vi "0037-Sub_map_meas.vi"(6 "数値":dbl, 7 "温湿度データ":dbl[][](array[numeric]), 8 "error out":errorcluster, 11 "device":T1) -> (0 "error out 2":errorcluster caption="error out", 2 "出力配列":dbl[](array[numeric]), 3 "device 2":T1, 4 "配列":bool[](array[boolean]), 5 "温湿度データ 2":dbl[][](array[numeric]))   [LabVIEW 2014]
uses:
  LV-CP2112_2014/LVProject/private/CP2112_device.ctl
  LV-CP2112_2014/LVProject/private/CP2112_SMBUS_S0.ctl
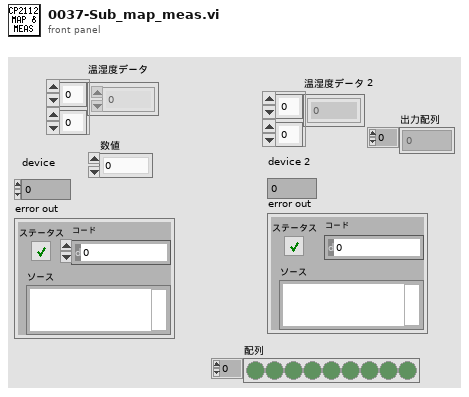
[diagram p1: front panel]
types:
  T1 = typedef "CP2112_device.ctl" = i32
  T2 = typedef "CP2112_SMBUS_S0.ctl" = enum8{"HID_SMBUS_S0_IDLE", "HID_SMBUS_S0_BUSY", "HID_SMBUS_S0_COMPLETE", "HID_SMBUS_S0_ERROR"}
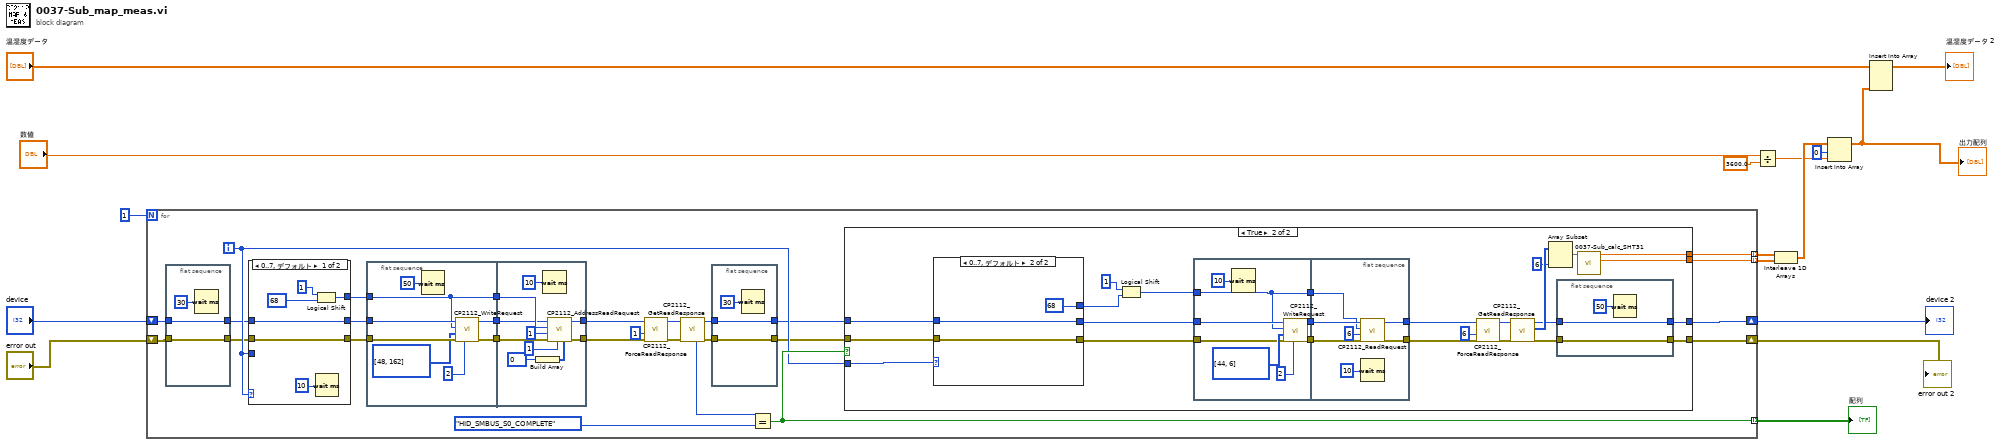
[diagram p0: block diagram]
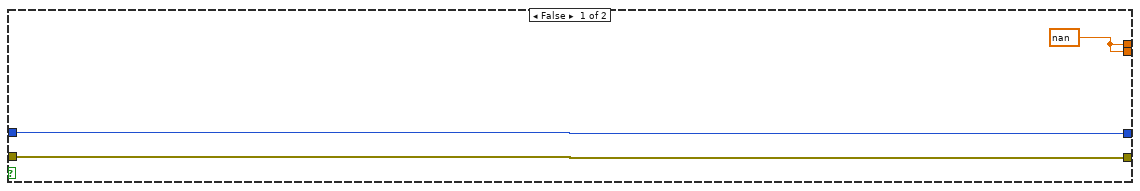
[diagram p2: hidden frame]
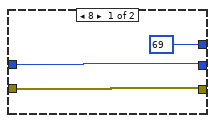
[diagram p3: hidden frame]
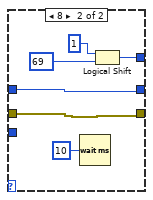
[diagram p4: hidden frame]
diagram:
  n1 = for {
    N: 1 -> [_]
    shift-right: [w28] -> w15
    shift-left: "error out" -> [w20]
    shift-right: [w29] -> w16
    shift-left: "device" -> [w19]
    tunnel: [w30] -> w13 mode=indexing
    tunnel: [w26] -> w8 mode=indexing
    tunnel: [w25] -> w7 mode=indexing
    i -> [w27]
    n2 = flat-sequence {
      tunnel: [w46] -> w18
      tunnel: w19 -> [w46]
      tunnel: [w45] -> w17
      tunnel: w20 -> [w45]
      frame #0 {
        n3 = Wait (ms)(milliseconds to wait=u32 30 ("ミリ秒待機時間")) -> ()  [unwired: 1 out]
      }
    }
    n4 = case shown="0..7, デフォルト" w27 {
      tunnel: [w123 w130] -> w36
      tunnel: w17 -> [w121 w127]
      tunnel: [w121 w127] -> w37
      tunnel: w18 -> [w120 w126]
      tunnel: [w120 w126] -> w38
      tunnel: w27 -> [_ _]
      frame 0..7, Default {
        n5 = Logical Shift(y=1, x=68) -> (x << y=w123:i32)
        n6 = Wait (ms)(milliseconds to wait=u32 10 ("ミリ秒待機時間")) -> ()  [unwired: 1 out]
      }
      frame 8 {
        n7 = Wait (ms)(milliseconds to wait=u32 10 ("ミリ秒待機時間")) -> ()  [unwired: 1 out]
        n8 = Logical Shift(y=1, x=69) -> (x << y=w130:i32)
      }
    }
    n9 = flat-sequence {
      tunnel: w38 -> [w109]
      tunnel: w37 -> [w107]
      tunnel: w36 -> [w105]
      tunnel: [w108] -> w35
      tunnel: [w106] -> w34
      tunnel: [w105] -> w33
      tunnel: w35 -> [w114]
      tunnel: w34 -> [w113]
      tunnel: w33 -> [w115]
      tunnel: [w112] -> w32
      tunnel: [w111] -> w31
      frame #0 {
        n10 = Wait (ms)(milliseconds to wait=u32 50 ("ミリ秒待機時間")) -> ()  [unwired: 1 out]
        n11 = call "CP2112_WriteRequest.vi"("numBytesToWrite"=u8 2, "error in (no error)"=w107, "buffer"=u8[] [48, 162], "slaveAddress"=w105, "device"=w109) -> ("error out"=w106:errorcluster, "deviceOut"=w108:T1)  [unwired: 4 in, 1 out]
      }
      frame #1 {
        n12 = Build Array(u8 0 ("targetAddressSize")) -> (w118:u8[])
        n13 = Wait (ms)(milliseconds to wait=u32 10 ("ミリ秒待機時間")) -> ()  [unwired: 1 out]
        n14 = call "CP2112_AddressReadRequest.vi"("targetAddress[]"=w118, "targetAddressSize"=u8 1, "error in (no error)"=w113, "numByteToRead"=i16 1, "slaveAddress"=w115, "device"=w114) -> ("error out"=w112:errorcluster, "deviceOut"=w111:T1)  [unwired: 3 in, 1 out]
      }
    }
    n15 = call "CP2112_ForceReadResponse.vi"("error in (no error)"=w32, "numByteToRead"=i16 1, "device"=w31) -> ("error out"=w43:errorcluster, "deviceOut"=w42:T1)  [unwired: 6 in, 1 out]
    n16 = call "CP2112_GetReadResponse.vi"("error in (no error)"=w43, "device"=w42) -> ("error out"=w21:errorcluster, "deviceOut"=w23:T1, "HID_SMBUS_S0"=w39:T2)  [unwired: 4 in, 3 out]
    n17 = flat-sequence {
      tunnel: [w49] -> w24
      tunnel: w23 -> [w49]
      tunnel: [w48] -> w22
      tunnel: w21 -> [w48]
      frame #0 {
        n18 = Wait (ms)(milliseconds to wait=u32 30 ("ミリ秒待機時間")) -> ()  [unwired: 1 out]
      }
    }
    n19 = Equal?(x=w39, y=CP2112_SMBUS_S0."HID_SMBUS_S0_COMPLETE" ("HID_SMBUS_S0")) -> (x = y?=w30:bool)
    n20 = case shown="TRUE" w30 {
      tunnel: [w51 w55] -> w28
      tunnel: [w52 w57] -> w29
      tunnel: w24 -> [w52 w72]
      tunnel: w22 -> [w51 w71]
      tunnel: w27 -> [_ w53]
      tunnel: [w50 w69] -> w26
      tunnel: [w50 w68] -> w25
      frame False {
        w50 = nan ("新規要素/部分配列")
      }
      frame True {
        n21 = case shown="0..7, デフォルト" w53 {
          tunnel: [w96 w100] -> w63
          tunnel: [w97 w99] -> w64
          tunnel: [u32 69 ("ミリ秒待機時間") u32 68 ("ミリ秒待機時間")] -> w66
          tunnel: w72 -> [w97 w99]
          tunnel: w71 -> [w96 w100]
          frame 8 {
          }
          frame 0..7, Default {
          }
        }
        n22 = Logical Shift(y=1, x=w66) -> (x << y=w65:u32)
        n23 = flat-sequence {
          tunnel: w65 -> [w82]
          tunnel: w64 -> [w84]
          tunnel: w63 -> [w83]
          tunnel: [w88] -> w62
          tunnel: [w87] -> w61
          tunnel: [w82] -> w58
          tunnel: w62 -> [w90]
          tunnel: w61 -> [w92]
          tunnel: [w94] -> w60
          tunnel: [w93] -> w59
          tunnel: w58 -> [w91]
          frame #0 {
            n24 = Wait (ms)(milliseconds to wait=u32 10 ("ミリ秒待機時間")) -> ()  [unwired: 1 out]
            n25 = call "CP2112_WriteRequest.vi"("numBytesToWrite"=i16 2 ("numByteToRead"), "error in (no error)"=w83, "buffer"=u8[] [44, 6], "slaveAddress"=w82, "device"=w84) -> ("error out"=w88:errorcluster, "deviceOut"=w87:T1)  [unwired: 4 in, 1 out]
          }
          frame #1 {
            n26 = call "CP2112_ReadRequest.vi"("error in (no error)"=w90, "numByteToRead"=i16 6, "slaveAddress"=w91, "device"=w92) -> ("error out"=w94:errorcluster, "deviceOut"=w93:T1)  [unwired: 5 in, 1 out]
            n27 = Wait (ms)(milliseconds to wait=u32 10 ("ミリ秒待機時間")) -> ()  [unwired: 1 out]
          }
        }
        n28 = call "CP2112_ForceReadResponse.vi"("error in (no error)"=w60, "numByteToRead"=i16 6, "device"=w59) -> ("error out"=w73:errorcluster, "deviceOut"=w74:T1)  [unwired: 6 in, 1 out]
        n29 = call "CP2112_GetReadResponse.vi"("error in (no error)"=w73, "device"=w74) -> ("error out"=w54:errorcluster, "buffer"=w77:u8[], "deviceOut"=w56:T1)  [unwired: 4 in, 3 out]
        n30 = Array Subset(array=w77, length=6 ("長さ")) -> (w75:u8[])  [unwired: 1 in]
        n31 = flat-sequence {
          tunnel: [w80] -> w57
          tunnel: w56 -> [w80]
          tunnel: [w79] -> w55
          tunnel: w54 -> [w79]
          frame #0 {
            n32 = Wait (ms)(milliseconds to wait=u32 50 ("ミリ秒待機時間")) -> ()  [unwired: 1 out]
          }
        }
        n33 = call "0037-Sub_calc_SHT31.vi"("Data"=w75) -> ("数値"=w68:dbl, "数値 2"=w69:dbl)  [unwired: 9 in]
      }
    }
  }
  "配列" <- w13
  "device 2" <- w16
  "error out 2" <- w15
  n34 = Divide(x="数値", y=3600.0) -> (x/y=w3:dbl)
  n35 = Interleave 1D Arrays(w8, w7) -> (w6:dbl[])
  n36 = Insert Into Array(array=w6, index=0 ("指標"), new element=w3) -> (w1:dbl[])
  "出力配列" <- w1
  n37 = Insert Into Array(array="温湿度データ", new element=w1) -> (→"温湿度データ 2":dbl[][])  [unwired: 2 in]
